vi "PCO_GetMetaDataExtern.vi"(8 "error in (no error)":errorcluster {"code" format="%x"}, 10 "pBuf":u16[][](array[numeric])=array1x4097[4097 elements], 11 "ph":u64) -> (0 "error out":errorcluster {"code" format="%x"}, 1 "MetaData":T1, 2 "ErrorMessage":i32 format="%x", 3 "ph out":u64)   [LabVIEW 2020, in "SDK.lvlib" / "RecordingControl.lvlib"]
doc: "<b>Description:</b>\nGets the image buffer attached meta data, if available\n\n<b>Supported camera type:</b>\nAll cameras\n\n<b>Descriptor dependency:</b>\nNone"
uses:
  RecordingControl.lvlib
  <vilib>/Utility/miscctls.llb/LVDateTimeRec.ctl
  Structures/Structures.lvlib
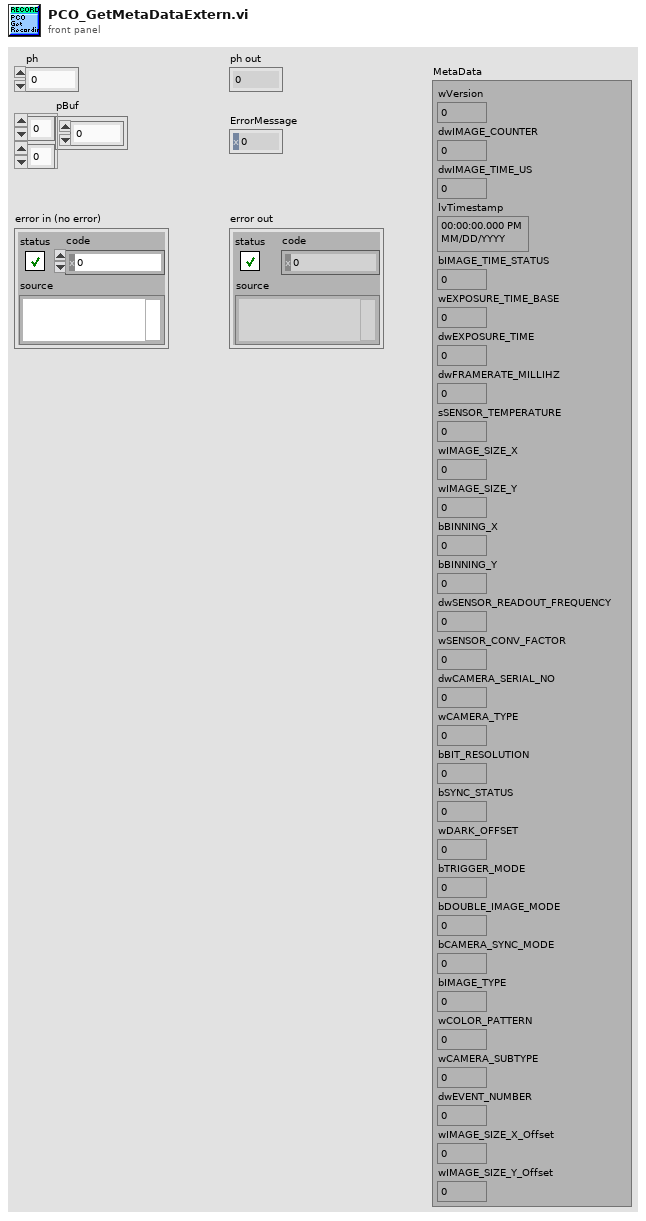
[diagram p1: front panel]
types:
  T1 = cluster{"wVersion":u16, "dwIMAGE_COUNTER":u32, "dwIMAGE_TIME_US":u32, "lvTimestamp":timestamp, "bIMAGE_TIME_STATUS":u8, "wEXPOSURE_TIME_BASE":u16, "dwEXPOSURE_TIME":u32, "dwFRAMERATE_MILLIHZ":u32, "sSENSOR_TEMPERATURE":i16, "wIMAGE_SIZE_X":u16, "wIMAGE_SIZE_Y":u16, "bBINNING_X":u8, "bBINNING_Y":u8, "dwSENSOR_READOUT_FREQUENCY":u32, "wSENSOR_CONV_FACTOR":u16, "dwCAMERA_SERIAL_NO":u32, "wCAMERA_TYPE":u16, "bBIT_RESOLUTION":u8, "bSYNC_STATUS":u8, "wDARK_OFFSET":u16, "bTRIGGER_MODE":u8, "bDOUBLE_IMAGE_MODE":u8, "bCAMERA_SYNC_MODE":u8, "bIMAGE_TYPE":u8, "wCOLOR_PATTERN":u16, "wCAMERA_SUBTYPE":u16, "dwEVENT_NUMBER":u32, "wIMAGE_SIZE_X_Offset":u16, "wIMAGE_SIZE_Y_Offset":u16}
  T2 = typedef "LVDateTimeRec.ctl" = cluster{"fractional second":dbl, "second":i32, "minute":i32, "hour":i32, "day of month":i32, "month":i32, "year":i32, "day of week":i32, "day of year":i32, "DST":i32}
  T3 = cluster{"wSize":u16, "wVersion":u16, "bIMAGE_COUNTER_BCD":cluster{u8, u8, u8, u8}, "bIMAGE_TIME_US_BCD":cluster{u8, u8, u8}, "bIMAGE_TIME_SEC_BCD":u8, "bIMAGE_TIME_MIN_BCD":u8, "bIMAGE_TIME_HOUR_BCD":u8, "bIMAGE_TIME_DAY_BCD":u8, "bIMAGE_TIME_MON_BCD":u8, "bIMAGE_TIME_YEAR_BCD":u8, "bIMAGE_TIME_STATUS":u8, "wEXPOSURE_TIME_BASE":u16, "dwEXPOSURE_TIME":u32, "dwFRAMERATE_MILLIHZ":u32, "sSENSOR_TEMPERATURE":i16, "wIMAGE_SIZE_X":u16, "wIMAGE_SIZE_Y":u16, "bBINNING_X":u8, "bBINNING_Y":u8, "dwSENSOR_READOUT_FREQUENCY":u32, "wSENSOR_CONV_FACTOR":u16, "dwCAMERA_SERIAL_NO":u32, "wCAMERA_TYPE":u16, "bBIT_RESOLUTION":u8, "bSYNC_STATUS":u8, "wDARK_OFFSET":u16, "bTRIGGER_MODE":u8, "bDOUBLE_IMAGE_MODE":u8, "bCAMERA_SYNC_MODE":u8, "bIMAGE_TYPE":u8, "wCOLOR_PATTERN":u16, "wCAMERA_SUBTYPE":u16, "dwEVENT_NUMBER":u32, "wIMAGE_SIZE_X_Offset":u16, "wIMAGE_SIZE_Y_Offset":u16}
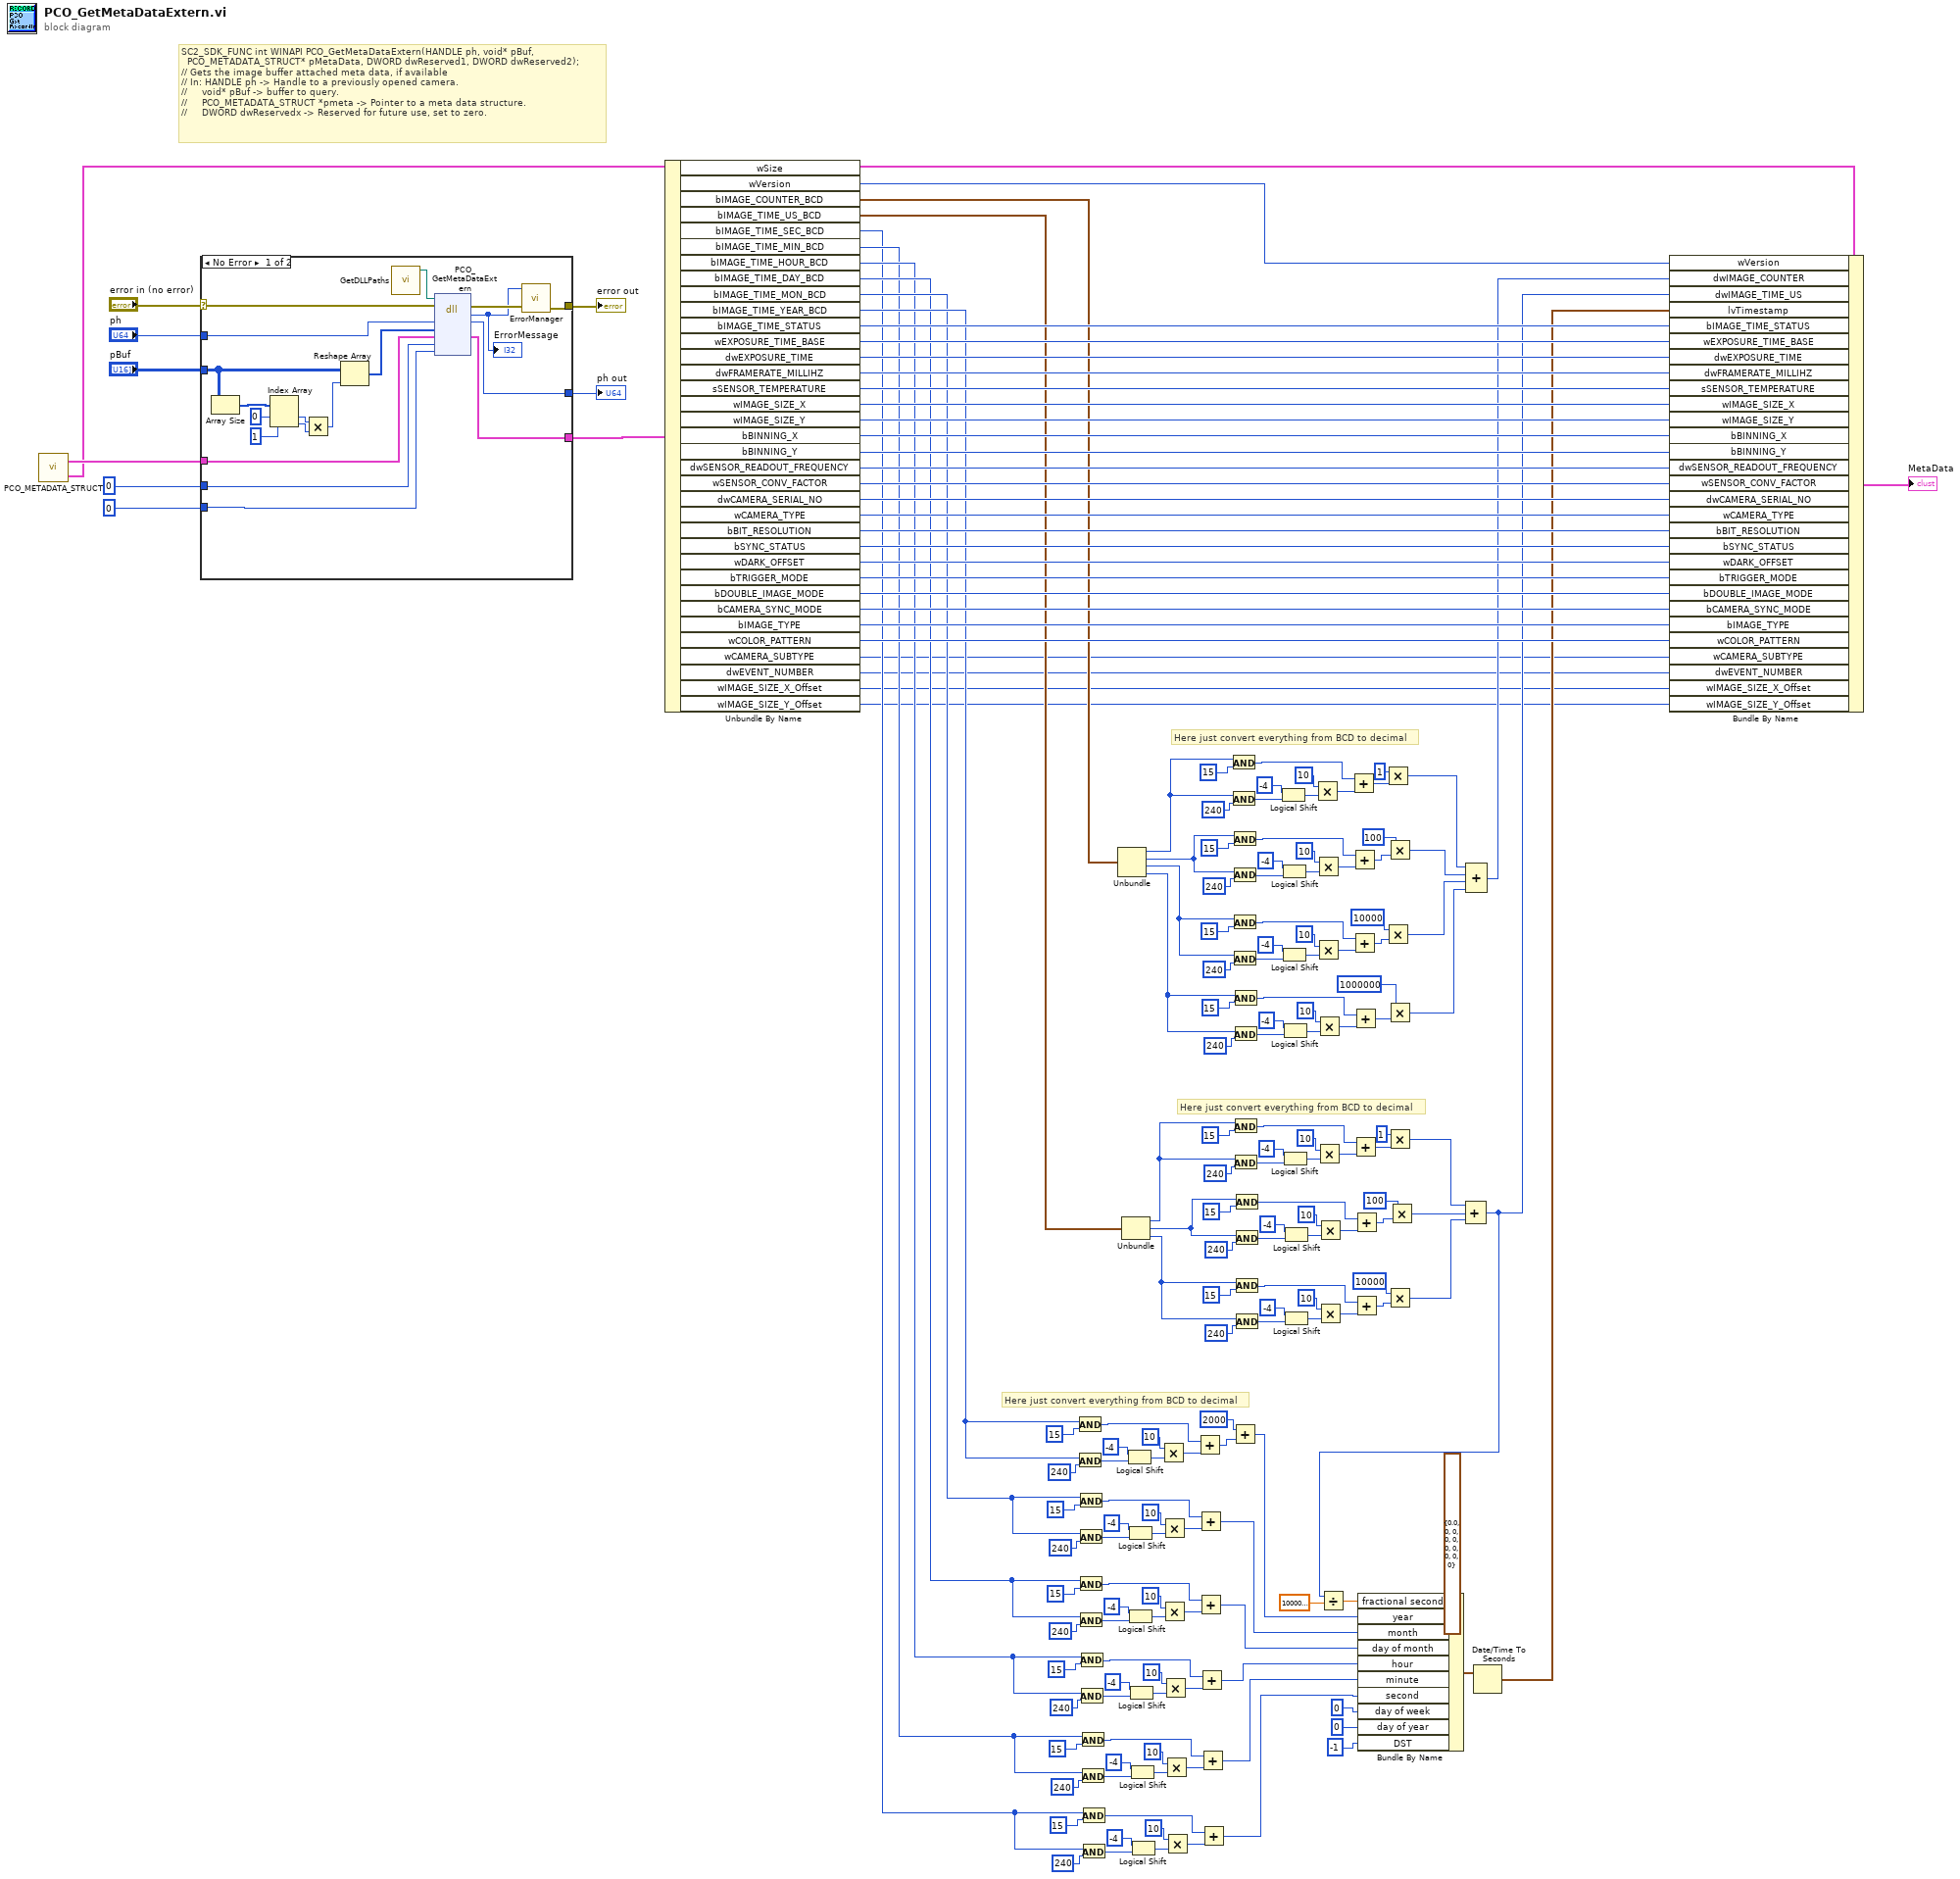
[diagram p0: block diagram]
diagram:
  # "Here just convert everything from BCD to decimal"
  # "Here just convert everything from BCD to decimal"
  # "Here just convert everything from BCD to decimal"
  # "SC2_SDK_FUNC int WINAPI PCO_GetMetaDataExtern(HANDLE ph, void* pBuf,\n  PCO_METADATA_STRUCT* pMetaData, DWORD dwReserved1, DWORD dwReserved2);\n// Gets the image buffer attached meta data, if available\n// In: HANDLE ph -> Handle to a previously opened camera.\n//     void* pBuf -> buffer to query.\n//     PCO_METADATA_STRUCT *pmeta -> Pointer to a meta data structure.\n//     DWORD dwReservedx -> Reserved for future use, set to zero."
  n1 = call "PCO_METADATA_STRUCT.vi"() -> ("PCO_METADATA_STRUCT"=w8:T1, "PCO_METADATA_STRUCT_Raw"=w191:T3)  [unwired: 4 in, 2 out]
  n2 = case shown="No Error" "error in (no error)" {
    selector: "error in (no error)" -> [w210 w217]
    tunnel: "ph" -> [w214 w216]
    tunnel: [w213 w216] -> w194
    tunnel: w191 -> [w212 w215]
    tunnel: [w211 w215] -> w7
    tunnel: [w208 w217] -> w193
    tunnel: u32 0 ("dwReserved1") -> [w205 _]
    tunnel: u32 0 ("dwReserved1") -> [w204 _]
    tunnel: "pBuf" -> [w198 _]
    frame No Error {
      n3 = Array Size(array=w198) -> (size(s)=w199:i32[])
      n4 = Index Array(array=w199, index #1=0 ("index"), index #2=1 ("index")) -> (element #1=w202:i32, element #2=w203:i32)
      n5 = Multiply(x=w202, y=w203) -> (x*y=w197:i32)
      n6 = Reshape Array(w198, w197) -> (w196:u16[])
      n7 = call "GetDLLPaths.vi"() -> ("SC2_Cam_Path"=w206:path)  [unwired: 9 in, 2 out]
      n8 = dll-call lib="?" fn="PCO_GetMetaDataExtern"(path in=w206, error in=w210, "ph"=w214, "pBuf"=w196, "pMetaData"=w212, "dwReserved1"=w205, "dwReserved2"=w204) -> (error out=w209:errorcluster, "return type"=w207:i32, "ph"=w213:u64, "pMetaData"=w211:T3)  [unwired: 4 in, 1 out]
      "ErrorMessage" <- w207
      n9 = call "ErrorManager.vi"("error in (no error)"=w209, "error code"=w207) -> ("error out"=w208:errorcluster)  [unwired: 3 in]
    }
    frame Error {
    }
  }
  "ph out" <- w194
  "error out" <- w193
  n10 = Unbundle By Name(w7) -> ("wVersion"=w188:u16, "bIMAGE_COUNTER_BCD"=w101:cluster{u8, u8, u8, u8}, "bIMAGE_TIME_US_BCD"=w23:cluster{u8, u8, u8}, "bIMAGE_TIME_SEC_BCD"=w113:u8, "bIMAGE_TIME_MIN_BCD"=w114:u8, "bIMAGE_TIME_HOUR_BCD"=w115:u8, "bIMAGE_TIME_DAY_BCD"=w116:u8, "bIMAGE_TIME_MON_BCD"=w117:u8, "bIMAGE_TIME_YEAR_BCD"=w162:u8, "bIMAGE_TIME_STATUS"=w184:u8, "wEXPOSURE_TIME_BASE"=w183:u16, "dwEXPOSURE_TIME"=w182:u32, "dwFRAMERATE_MILLIHZ"=w181:u32, "sSENSOR_TEMPERATURE"=w180:i16, "wIMAGE_SIZE_X"=w179:u16, "wIMAGE_SIZE_Y"=w178:u16, "bBINNING_X"=w177:u8, "bBINNING_Y"=w176:u8, "dwSENSOR_READOUT_FREQUENCY"=w175:u32, "wSENSOR_CONV_FACTOR"=w174:u16, "dwCAMERA_SERIAL_NO"=w173:u32, "wCAMERA_TYPE"=w172:u16, "bBIT_RESOLUTION"=w171:u8, "bSYNC_STATUS"=w170:u8, "wDARK_OFFSET"=w169:u16, "bTRIGGER_MODE"=w168:u8, "bDOUBLE_IMAGE_MODE"=w167:u8, "bCAMERA_SYNC_MODE"=w166:u8, "bIMAGE_TYPE"=w165:u8, "wCOLOR_PATTERN"=w164:u16, "wCAMERA_SUBTYPE"=w5:u16, "dwEVENT_NUMBER"=w4:u32, "wIMAGE_SIZE_X_Offset"=w3:u16, "wIMAGE_SIZE_Y_Offset"=w2:u16)  [unwired: 1 out]
  n11 = And(x=w162, y=u8 15) -> (x .and. y?=w158:u8)
  n12 = And(x=w162, y=u8 240) -> (x .and. y?=w185:u8)
  n13 = And(x=w117, y=u8 15) -> (x .and. y?=w157:u8)
  n14 = And(x=w117, y=u8 240) -> (x .and. y?=w152:u8)
  n15 = And(x=w116, y=u8 15) -> (x .and. y?=w141:u8)
  n16 = And(x=w116, y=u8 240) -> (x .and. y?=w136:u8)
  n17 = And(x=w115, y=u8 15) -> (x .and. y?=w142:u8)
  n18 = And(x=w115, y=u8 240) -> (x .and. y?=w147:u8)
  n19 = And(x=w114, y=u8 15) -> (x .and. y?=w126:u8)
  n20 = And(x=w114, y=u8 240) -> (x .and. y?=w131:u8)
  n21 = And(x=w113, y=u8 15) -> (x .and. y?=w125:u8)
  n22 = And(x=w113, y=u8 240) -> (x .and. y?=w120:u8)
  n23 = Unbundle(w101) -> (w31:u8, w30:u8, w29:u8, w28:u8)
  n24 = Unbundle(w23) -> (w22:u8, w21:u8, w20:u8)
  n25 = Logical Shift(y=i16 -4, x=w185) -> (x << y=w161:u8)
  n26 = Logical Shift(y=i16 -4, x=w152) -> (x << y=w154:u8)
  n27 = Logical Shift(y=i16 -4, x=w136) -> (x << y=w138:u8)
  n28 = Logical Shift(y=i16 -4, x=w147) -> (x << y=w145:u8)
  n29 = Logical Shift(y=i16 -4, x=w131) -> (x << y=w129:u8)
  n30 = Logical Shift(y=i16 -4, x=w120) -> (x << y=w122:u8)
  n31 = Multiply(x=u8 10, y=w161) -> (x*y=w159:u8)
  n32 = Multiply(x=u8 10, y=w154) -> (x*y=w156:u8)
  n33 = Multiply(x=u8 10, y=w138) -> (x*y=w140:u8)
  n34 = Multiply(x=u8 10, y=w145) -> (x*y=w143:u8)
  n35 = Multiply(x=u8 10, y=w129) -> (x*y=w127:u8)
  n36 = Multiply(x=u8 10, y=w122) -> (x*y=w124:u8)
  n37 = Add(x=w158, y=w159) -> (x+y=w14:u8)
  n38 = Add(x=w157, y=w156) -> (x+y=w107:u8)
  n39 = Add(x=w141, y=w140) -> (x+y=w106:u8)
  n40 = Add(x=w142, y=w143) -> (x+y=w105:u8)
  n41 = Add(x=w126, y=w127) -> (x+y=w104:u8)
  n42 = Add(x=w125, y=w124) -> (x+y=w103:u8)
  n43 = And(x=w31, y=u8 15) -> (x .and. y?=w76:u8)
  n44 = And(x=w31, y=u8 240) -> (x .and. y?=w71:u8)
  n45 = And(x=w30, y=u8 15) -> (x .and. y?=w77:u8)
  n46 = And(x=w30, y=u8 240) -> (x .and. y?=w82:u8)
  n47 = And(x=w29, y=u8 15) -> (x .and. y?=w93:u8)
  n48 = And(x=w29, y=u8 240) -> (x .and. y?=w98:u8)
  n49 = Add(x=2000, y=w14) -> (x+y=w12:i32)
  n50 = And(x=w28, y=u8 15) -> (x .and. y?=w92:u8)
  n51 = And(x=w28, y=u8 240) -> (x .and. y?=w87:u8)
  n52 = And(x=w22, y=u8 15) -> (x .and. y?=w47:u8)
  n53 = And(x=w22, y=u8 240) -> (x .and. y?=w52:u8)
  n54 = And(x=w21, y=u8 15) -> (x .and. y?=w46:u8)
  n55 = And(x=w21, y=u8 240) -> (x .and. y?=w41:u8)
  n56 = And(x=w20, y=u8 15) -> (x .and. y?=w38:u8)
  n57 = And(x=w20, y=u8 240) -> (x .and. y?=w33:u8)
  n58 = Logical Shift(y=i16 -4, x=w71) -> (x << y=w73:u8)
  n59 = Logical Shift(y=i16 -4, x=w82) -> (x << y=w80:u8)
  n60 = Logical Shift(y=i16 -4, x=w98) -> (x << y=w96:u8)
  n61 = Logical Shift(y=i16 -4, x=w87) -> (x << y=w89:u8)
  n62 = Logical Shift(y=i16 -4, x=w52) -> (x << y=w50:u8)
  n63 = Logical Shift(y=i16 -4, x=w41) -> (x << y=w43:u8)
  n64 = Logical Shift(y=i16 -4, x=w33) -> (x << y=w35:u8)
  n65 = Multiply(x=u8 10, y=w73) -> (x*y=w75:u8)
  n66 = Multiply(x=u8 10, y=w80) -> (x*y=w78:u8)
  n67 = Multiply(x=u8 10, y=w96) -> (x*y=w94:u8)
  n68 = Multiply(x=u8 10, y=w89) -> (x*y=w91:u8)
  n69 = Multiply(x=u8 10, y=w50) -> (x*y=w48:u8)
  n70 = Multiply(x=u8 10, y=w43) -> (x*y=w45:u8)
  n71 = Multiply(x=u8 10, y=w35) -> (x*y=w37:u8)
  n72 = Add(x=w76, y=w75) -> (x+y=w65:u8)
  n73 = Add(x=w77, y=w78) -> (x+y=w68:u8)
  n74 = Add(x=w93, y=w94) -> (x+y=w67:u8)
  n75 = Add(x=w92, y=w91) -> (x+y=w66:u8)
  n76 = Add(x=w47, y=w48) -> (x+y=w57:u8)
  n77 = Add(x=w46, y=w45) -> (x+y=w55:u8)
  n78 = Add(x=w38, y=w37) -> (x+y=w56:u8)
  n79 = Multiply(x=u32 1, y=w65) -> (x*y=w27:u32)
  n80 = Multiply(x=u32 10000, y=w67) -> (x*y=w25:u32)
  n81 = Multiply(x=u32 100, y=w68) -> (x*y=w26:u32)
  n82 = Multiply(x=u32 1000000, y=w66) -> (x*y=w24:u32)
  n83 = Multiply(x=u32 1, y=w57) -> (x*y=w18:u32)
  n84 = Multiply(x=u32 10000, y=w56) -> (x*y=w16:u32)
  n85 = Multiply(x=u32 100, y=w55) -> (x*y=w17:u32)
  n86 = Compound Arithmetic op=ADD(w18, w17, w16) -> (w10:u32)
  n87 = Divide(x=w10, y=1000000.0 ("fractional second")) -> (x/y=w9:dbl)
  n88 = Bundle By Name(cluster=T2 {"fractional second"=0.0, "second"=0, "minute"=0, "hour"=0, "day of month"=0, "month"=0, "year"=0, "day of week"=0, "day of year"=0, "DST"=0} ("date time rec"), "fractional second"=w9, "year"=w12, "month"=w107, "day of month"=w106, "hour"=w105, "minute"=w104, "second"=w103, "day of week"=0, "day of year"=0, "DST"=-1) -> (w108:T2)
  n89 = Compound Arithmetic op=ADD(w27, w26, w25, w24) -> (w15:u32)
  n90 = Date/Time To Seconds(2:w108) -> (0:w102:timestamp)  [unwired: 1 in]
  n91 = Bundle By Name(cluster=w8, "wVersion"=w188, "dwIMAGE_COUNTER"=w15, "dwIMAGE_TIME_US"=w10, "lvTimestamp"=w102, "bIMAGE_TIME_STATUS"=w184, "wEXPOSURE_TIME_BASE"=w183, "dwEXPOSURE_TIME"=w182, "dwFRAMERATE_MILLIHZ"=w181, "sSENSOR_TEMPERATURE"=w180, "wIMAGE_SIZE_X"=w179, "wIMAGE_SIZE_Y"=w178, "bBINNING_X"=w177, "bBINNING_Y"=w176, "dwSENSOR_READOUT_FREQUENCY"=w175, "wSENSOR_CONV_FACTOR"=w174, "dwCAMERA_SERIAL_NO"=w173, "wCAMERA_TYPE"=w172, "bBIT_RESOLUTION"=w171, "bSYNC_STATUS"=w170, "wDARK_OFFSET"=w169, "bTRIGGER_MODE"=w168, "bDOUBLE_IMAGE_MODE"=w167, "bCAMERA_SYNC_MODE"=w166, "bIMAGE_TYPE"=w165, "wCOLOR_PATTERN"=w164, "wCAMERA_SUBTYPE"=w5, "dwEVENT_NUMBER"=w4, "wIMAGE_SIZE_X_Offset"=w3, "wIMAGE_SIZE_Y_Offset"=w2) -> (→"MetaData":T1)
